vi "UDPrecieverNoLoop.vi"() -> ()   [LabVIEW 2012]
panel:
  out "Profile":u32[](graph)
  in  "Profile Number":u32=1
  out "Profile Byte by Byte":u8[](graph)
  out "Header Array":bool[][](array[boolean])
  out "NumBins":u32
  out "Cnts/Bin":u32
  out "Prof/Hist":u32
  out "Sync":u32
  out "Channel":u32
  out "rTime":u32
  out "frameCntr":u32
  out "built packet array":string[](array[string])
  out "error post-check":errorcluster
  out "End Reciever Error":errorcluster
  in  "stop reciever":bool
  out "port":u16
  out "error out post-read":errorcluster
  out "error out pre-read":errorcluster
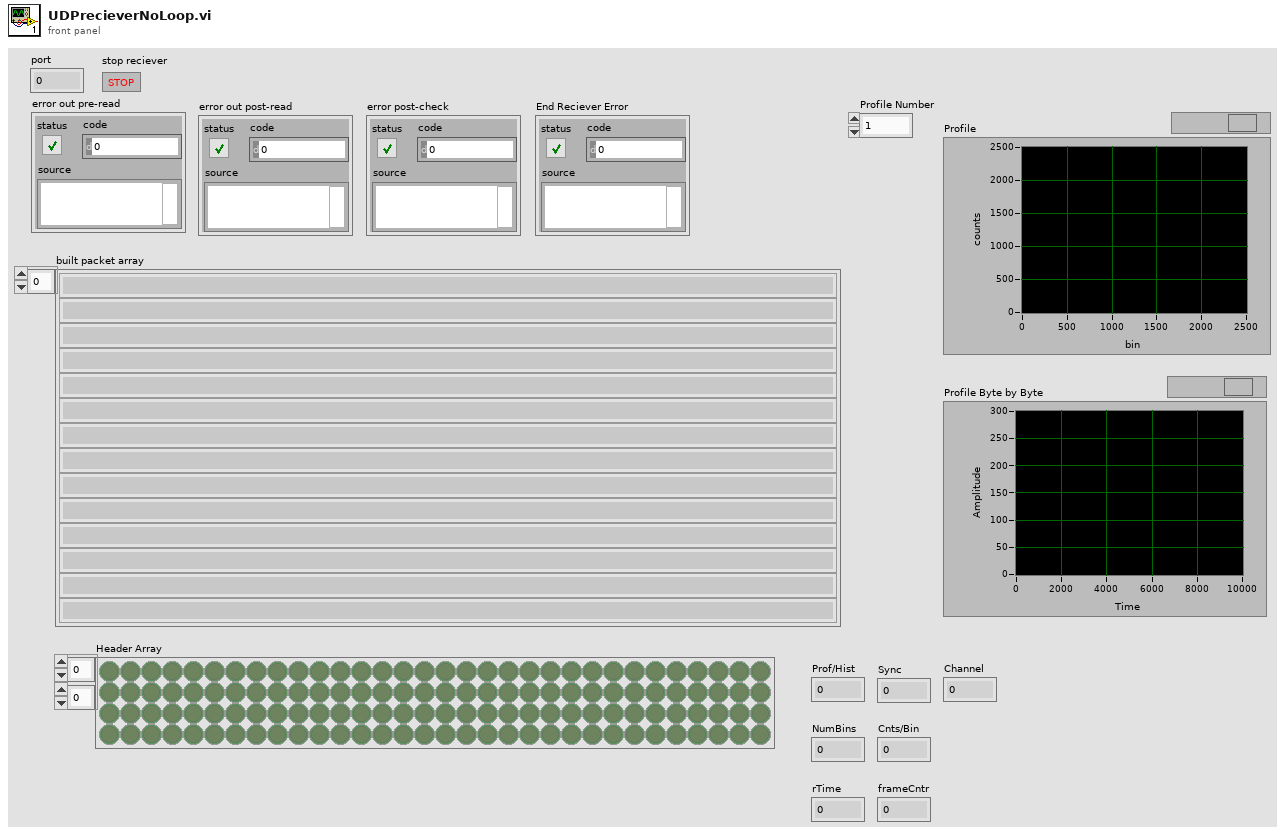
[diagram p1: front panel]
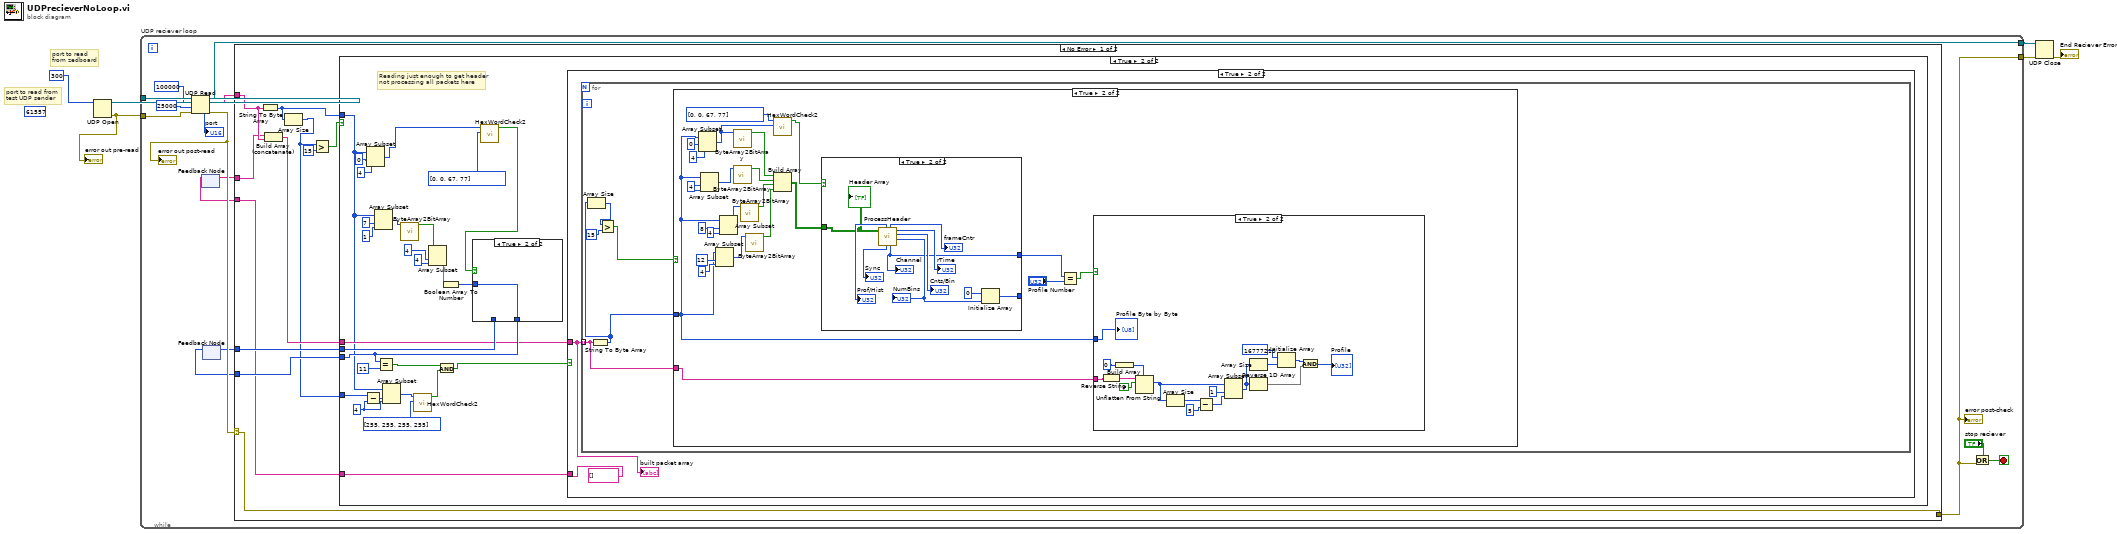
[diagram p0: block diagram]
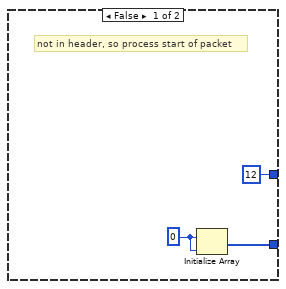
[diagram p6: hidden frame]
diagram:
  (unwired) u16 61557 ("port")
  # "port to read \nfrom zedboard"
  # "port to read from \ntest UDP sender"
  n1 = UDP Open(11:u16 300 ("port")) -> (port=w5:refnum<k16>, 0:w2:errorcluster)  [unwired: 4 in, 1 out]
  "error out pre-read" <- w2
  n2 = while "UDP reciever loop" {
    tunnel: [w21] -> w6
    tunnel: w5 -> [w20]
    tunnel: [w12] -> w4
    tunnel: w2 -> [w17]
    stop <- w19 stop-if-true
    n3 = UDP Read(connection ID=w20, max size (548)=100000, timeout ms (25000)=25000, 8:w17) -> (data out=w14:string, error out=w16:errorcluster, 3:w21:refnum<k16>, 4:→"port":u16)  [unwired: 1 out]
    "error out post-read" <- w16
    n4 = feedback #1() -> (w9:string[])  [unwired: 1 in]
    n5 = feedback #2() -> (w7:u32)  [unwired: 1 in]
    n6 = case shown="No Error" w16 {
      selector: w16 -> [w32 w127]
      tunnel: w14 -> [w31 _]
      tunnel: [w32 w127] -> w12
      tunnel: [w23 w126] -> w10
      tunnel: w9 -> [w30 w126]
      tunnel: [w27 w125] -> w8
      tunnel: w7 -> [w26 w125]
      frame No Error {
        n7 = String To Byte Array(string=w31) -> (unsigned byte array=w24:u8[])
        n8 = Build Array (concatenate)(w30, w31) -> (w25:string[])
        n9 = Array Size(array=w24) -> (size(s)=w22:i32)
        n10 = Greater?(x=w22, y=15) -> (0:w29:bool)
        n11 = case shown="True" w29 {
          tunnel: w24 -> [_ w44]
          tunnel: [w34 w48] -> w27
          tunnel: w26 -> [w34 w49]
          tunnel: w22 -> [_ w52]
          tunnel: w25 -> [w33 w46]
          tunnel: [w33 w45] -> w23
          frame False {
          }
          frame True {
            w54 = 4 ("length")
            # "Reading just enough to get header\nnot processing all packets here"
            n12 = Subtract(x=w52, y=w54) -> (x-y=w53:i32)
            n13 = Array Subset(array=w44, index=0, length=4) -> (w58:u8[])
            n14 = Array Subset(array=w44, index=7, length=1) -> (w41:u8[])
            n15 = Array Subset(array=w44, index=w53, length=w54) -> (w47:u8[])
            n16 = call "ByteArray2BitArray.vi"("array"=w41) -> ("Array"=w38:bool[])  [unwired: 10 in]
            n17 = call "HexWordCheck2.vi"("array"=u8[] [255, 255, 255, 255], "Input Array"=w47) -> ("Boolean"=w55:bool)  [unwired: 9 in]
            n18 = Array Subset(array=w38, index=4, length=4) -> (w36:bool[])
            n19 = Boolean Array To Number(Boolean array=w36) -> (number=w37:u32)
            n20 = call "HexWordCheck2.vi"("array"=u8[] [0, 0, 67, 77], "Input Array"=w58) -> ("Boolean"=w35:bool)  [unwired: 9 in]
            n21 = case shown="True" w35 {
              tunnel: [w123 w124] -> w48
              tunnel: w49 -> [w123 _]
              tunnel: w37 -> [_ w124]
              frame False {
              }
              frame True {
              }
            }
            n22 = Equal?(x=w48, y=u32 11) -> (x = y?=w51:bool)
            n23 = And(x=w51, y=w55) -> (x .and. y?=w56:bool)
            n24 = case shown="True" w56 {
              tunnel: w46 -> [w62 w63]
              tunnel: [w62 string[] []] -> w45
              frame False {
              }
              frame True {
                n25 = for {
                  tunnel: w63 -> [w65] mode=indexing
                  n26 = String To Byte Array(string=w65) -> (unsigned byte array=w69:u8[])
                  n27 = Array Size(array=w69) -> (size(s)=w68:i32)
                  n28 = Greater?(x=w68, y=15) -> (0:w66:bool)
                  n29 = case shown="True" w66 {
                    tunnel: w69 -> [_ w72]
                    tunnel: w65 -> [_ w71]
                    frame False {
                    }
                    frame True {
                      w81 = 4 ("length")
                      n30 = Array Subset(array=w72, index=0, length=4) -> (w91:u8[])
                      n31 = Array Subset(array=w72, index=w81, length=w81) -> (w77:u8[])
                      n32 = Array Subset(array=w72, index=12, length=4) -> (w90:u8[])
                      n33 = Array Subset(array=w72, index=8, length=4) -> (w78:u8[])
                      n34 = call "ByteArray2BitArray.vi"("array"=w77) -> ("Array"=w87:bool[])  [unwired: 10 in]
                      n35 = call "ByteArray2BitArray.vi"("array"=w91) -> ("Array"=w86:bool[])  [unwired: 10 in]
                      n36 = call "ByteArray2BitArray.vi"("array"=w78) -> ("Array"=w89:bool[])  [unwired: 10 in]
                      n37 = call "ByteArray2BitArray.vi"("array"=w90) -> ("Array"=w88:bool[])  [unwired: 10 in]
                      n38 = call "HexWordCheck2.vi"("array"=w91, "Input Array"=u8[] [0, 0, 67, 77] ("array")) -> ("Boolean"=w76:bool)  [unwired: 9 in]
                      n39 = Build Array(w86, w87, w89, w88) -> (w75:bool[][])
                      n40 = case shown="True" w76 {
                        tunnel: w75 -> [_ w116]
                        tunnel: [w112 w113] -> _
                        tunnel: [u32 12 ("Numeric 4") w114] -> w74
                        frame False {
                          w110 = u32 0 ("element")
                          # "not in header, so process start of packet"
                          n41 = Initialize Array(w110, w110) -> (w112:u32[])
                        }
                        frame True {
                          n42 = call "ProcessHeader.vi"("Array"=w116) -> ("Numeric"=w117:u32, "Numeric 7"=→"Cnts/Bin":u32, "Numeric 3"=→"rTime":u32, "Numeric 4"=w114:u32, "Numeric 2"=→"frameCntr":u32, "Numeric 5"=→"Sync":u32, "Numeric 6"=→"Prof/Hist":u32)  [unwired: 4 in]
                          "NumBins" <- w117
                          "Channel" <- w114
                          n43 = Initialize Array(u32 0 ("element"), w117) -> (w113:u32[])
                          "Header Array" <- w116
                        }
                      }
                      n44 = Equal?(x=w74, y="Profile Number") -> (x = y?=w73:bool)
                      n45 = case shown="True" w73 {
                        tunnel: w72 -> [_ w109]
                        tunnel: w71 -> [_ w100]
                        frame False {
                        }
                        frame True {
                          n46 = Reverse String(1:w100) -> (0:w99:string)
                          n47 = Build Array(u32 0) -> (w107:u32[])
                          n48 = Unflatten From String(type=w107, binary string=w99, data includes array or string size? (T)=FALSE) -> (value=w105:u32[])  [unwired: 2 in, 2 out]
                          n49 = Array Size(array=w105) -> (size(s)=w104:i32)
                          n50 = Subtract(x=w104, y=5) -> (x-y=w101:i32)
                          n51 = Array Subset(array=w105, index=1, length=w101) -> (w98:u32[])
                          n52 = Reverse 1D Array(array=w98) -> (reversed array=w97:u32[])
                          n53 = Array Size(array=w98) -> (size(s)=w95:i32)
                          n54 = Initialize Array(u32 16777215 ("x*2^n"), w95) -> (w96:u32[])
                          n55 = And(x=w96, y=w97) -> (x .and. y?=→"Profile":u32[])
                          "Profile Byte by Byte" <- w109
                        }
                      }
                    }
                  }
                }
                "built packet array" <- w63
              }
            }
          }
        }
      }
      frame Error {
      }
    }
    "error post-check" <- w12
    n56 = feedback-in #1(w10) -> ()
    n57 = feedback-in #2(w8) -> ()
    n58 = Or(x="stop reciever", y=w12) -> (x .or. y?=w19:bool)
  }
  n59 = UDP Close(connection ID=w6, 8:w4) -> (error out=→"End Reciever Error":errorcluster)  [unwired: 1 out]
